vi "XSens DT Scan (SubVI).vi"(0 "string in":string, 1 "Index":i16, 2 "Payload Size":i16, 3 "Error In":errorcluster) -> (5 "DT Out":string[](array[string]), 6 "DT String":string[](array[string]), 8 "Error Out":errorcluster)   [LabVIEW 2019]
doc: "Parses the XSens data packet and outputs the data types, measurement strings, data type byte counts, and index (or offset) to start of each data measurment string in arrays. \n\n2020 NREL"
panel:
  out "Index Out":i16[](array[numeric])
  out "DT Size":u8[](array[numeric])
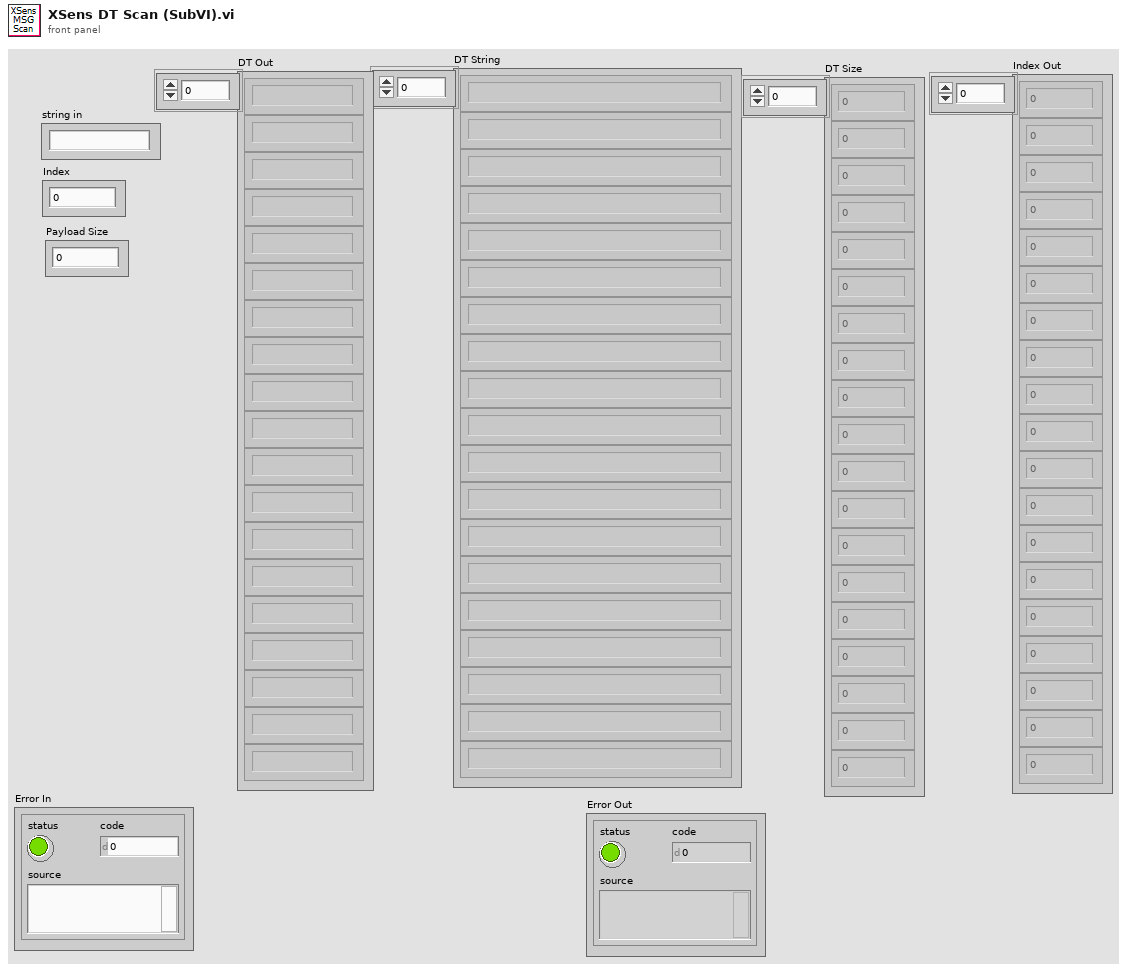
[diagram p1: front panel]
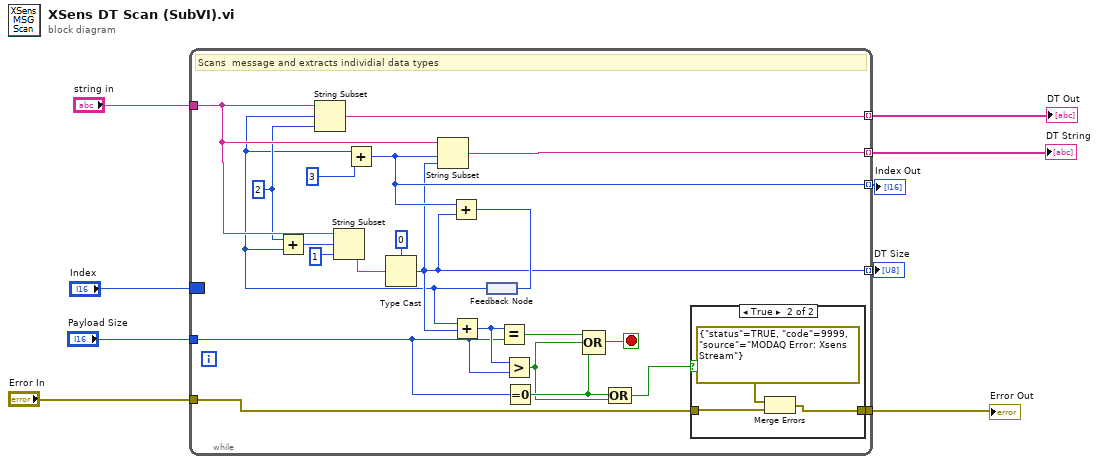
[diagram p0: block diagram]
diagram:
  n1 = while {
    tunnel: [w19] -> w7 mode=indexing
    tunnel: [w31] -> w9 mode=indexing
    tunnel: "string in" -> [w30]
    tunnel: [w29] -> w8 mode=indexing
    tunnel: [w21] -> w6 mode=indexing
    tunnel: "Payload Size" -> [w15]
    border: "Index" -> [_]
    tunnel: "Error In" -> [w11]
    tunnel: [w10] -> w1
    stop <- w16 stop-if-true
    w24 = 2 ("length (rest)")
    # "Scans  message and extracts individial data types"
    n2 = feedback #1() -> (w18:i16)
    n3 = Add(x=w24, y=w18) -> (x+y=w25:i32)
    n4 = String Subset(string=w30, offset (0)=w18, length (rest)=w24) -> (substring=w29:string)
    n5 = String Subset(string=w30, offset (0)=w25, length (rest)=1 ("length (rest)")) -> (substring=w27:string)
    n6 = Add(x=w18, y=i16 3) -> (x+y=w21:i16)
    n7 = Type Cast(type=u8 0, x=w27) -> (*(type *) &x=w19:u8)
    n8 = String Subset(string=w30, offset (0)=w21, length (rest)=w19) -> (substring=w31:string)
    n9 = Add(x=w21, y=w19) -> (x+y=w20:i16)
    n10 = Add(x=w18, y=w19) -> (x+y=w17:i16)
    n11 = feedback-in #1(w20) -> ()
    n12 = Equal?(x=w17, y=w15) -> (x = y?=w22:bool)
    n13 = Greater?(x=w17, y=w15) -> (0:w13:bool)
    n14 = Equal To 0?(x=w15) -> (x = 0?=w14:bool)
    n15 = Compound Arithmetic op=OR(w22, w13, w14) -> (w16:bool)
    n16 = Compound Arithmetic op=OR(w14, w13) -> (w12:bool)
    n17 = case shown="True" w12 {
      tunnel: w11 -> [w32 w35]
      tunnel: [w32 w34] -> w10
      frame False {
      }
      frame True {
        n18 = Merge Errors(errorcluster {"status"=TRUE, "code"=9999, "source"="MODAQ Error: Xsens Stream"} ("error in"), w35) -> (w34:errorcluster)
      }
    }
  }
  "Index Out" <- w6
  "DT Size" <- w7
  "DT Out" <- w8
  "DT String" <- w9
  "Error Out" <- w1
